vi "GFITS_CheckDir.vi"(4 "create?":bool=TRUE, 8 "error in":errorcluster, 11 "impath in":path) -> (0 "error out":errorcluster, 3 "impath out":path)   [LabVIEW 2016]
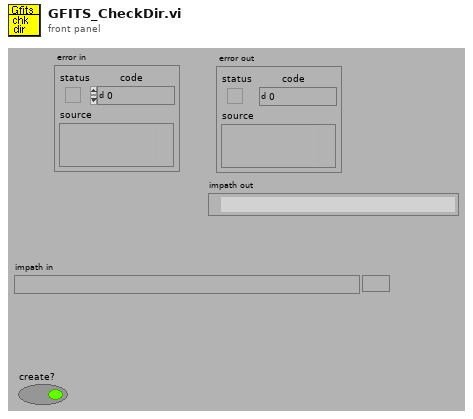
[diagram p1: front panel]
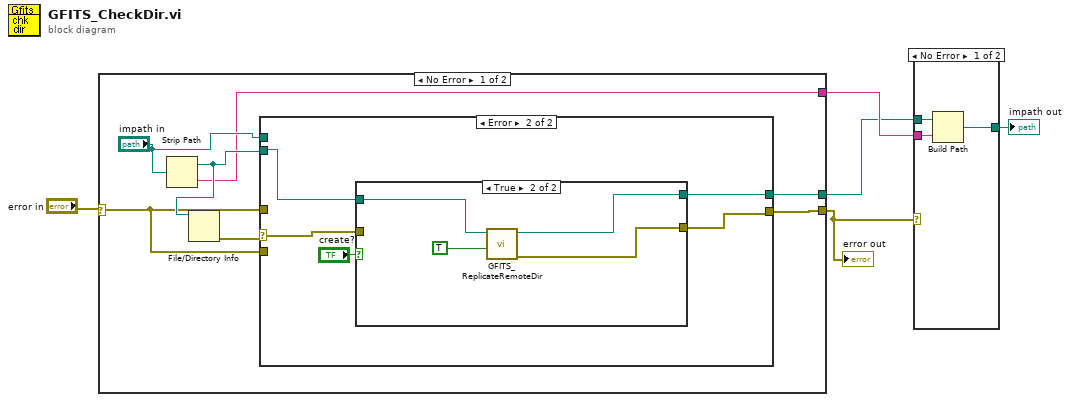
[diagram p0: block diagram]
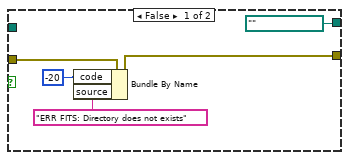
[diagram p4: hidden frame]
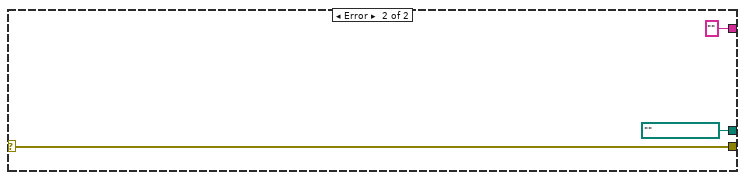
[diagram p5: hidden frame]
diagram:
  n1 = case shown="No Error" "error in" {
    selector: "error in" -> [w9 w31]
    tunnel: [w12 w31] -> w4
    tunnel: [w8 path "" ("local dir  out")] -> w2
    tunnel: [w6 "" ("name")] -> w3
    frame No Error {
      n2 = Strip Path(path="impath in") -> (stripped path=w10:path, name=w6:string)
      n3 = File/Directory Info(path=w10) -> (error out=w11:errorcluster)  [unwired: 1 in, 6 out]
      n4 = case shown="Error" w11 {
        selector: w11 -> [_ w19]
        tunnel: [w14 w18] -> w12
        tunnel: w9 -> [w14 _]
        tunnel: w10 -> [w13 w17]
        tunnel: w9 -> [_ _]
        tunnel: [w13 w16] -> w8
        tunnel: "impath in" -> [_ _]
        frame No Error {
        }
        frame Error {
          n5 = case shown="True" "create?" {
            tunnel: w19 -> [w24 _]
            tunnel: [w23 w28] -> w18
            tunnel: w17 -> [_ w27]
            tunnel: [path "" ("local dir  out") w25] -> w16
            frame False {
              n6 = Bundle By Name(cluster=w24, "code"=-20, "source"="ERR FITS: Directory does not exists") -> (w23:errorcluster)
            }
            frame True {
              n7 = call "GFITS_ReplicateRemoteDir.vi"("replicate remote dir?"=TRUE, "remote dir"=w27) -> ("error"=w28:errorcluster, "local dir  out"=w25:path)  [unwired: 2 in, 5 out]
            }
          }
        }
      }
    }
    frame Error {
    }
  }
  "error out" <- w4
  n8 = case shown="No Error" w4 {
    tunnel: w3 -> [w34 _]
    tunnel: w2 -> [w33 w35]
    tunnel: [w32 w35] -> w1
    frame No Error {
      n9 = Build Path(base path=w33, name or relative path=w34) -> (appended path=w32:path)
    }
    frame Error {
    }
  }
  "impath out" <- w1
